vi "TSLIN_LIN_Schedule_add.vi"(8 "错误输入":errorcluster, 10 "LIN Scheduling Table Array":T1[](array[typedef]) {"LIN_Transmit"."FDatas"."value 7" format="%.0x"; "LIN_Transmit"."FDatas"."value 6" format="%.0x"; "LIN_Transmit"."FDatas"."value 5" format="%.0x"; "LIN_Transmit"."FDatas"."value 4" format="%.0x"; "LIN_Transmit"."FDatas"."value 3" format="%.0x"; "LIN_Transmit"."FDatas"."value 2" format="%.0x"; "LIN_Transmit"."FDatas"."value 1" format="%.0x"; "LIN_Transmit"."FDatas"."value0" format="%.0x"; "LIN_Transmit"."Channel" items=["CHN1", "CHN2", "CHN3", "CHN4", "CHN5", "CHN6", "CHN7", "CHN8", "CHN9", "CHN10", "CHN11", "CHN12", "CHN13", "CHN14", "CHN15", "CHN16", "CHN17", "CHN18", "CHN19", "CHN20", "CHN21", "CHN22", "CHN23", "CHN24", "CHN25", "CHN26", "CHN27", "CHN28", "CHN29", "CHN30", "CHN31", "CHN32"]; "LIN_Transmit"."ID" format="%.0x"; "LIN_Transmit"."DLC" format="%.0x"; "LIN_Transmit"."Set_node_funtiontype" items=["MasterNode", "SlaveNode", "MonitorNote"]}, 11 "路径输入":path) -> (0 "错误输出":errorcluster, 1 "Channel array":i32[](array[numeric]), 2 "Successful?":bool, 3 "路径输出":path)   [LabVIEW 2014]
uses:
  Typedef/TSLIN_Transmit.ctl
  Typedef/TSLIN_LIN Schedule_Table.ctl
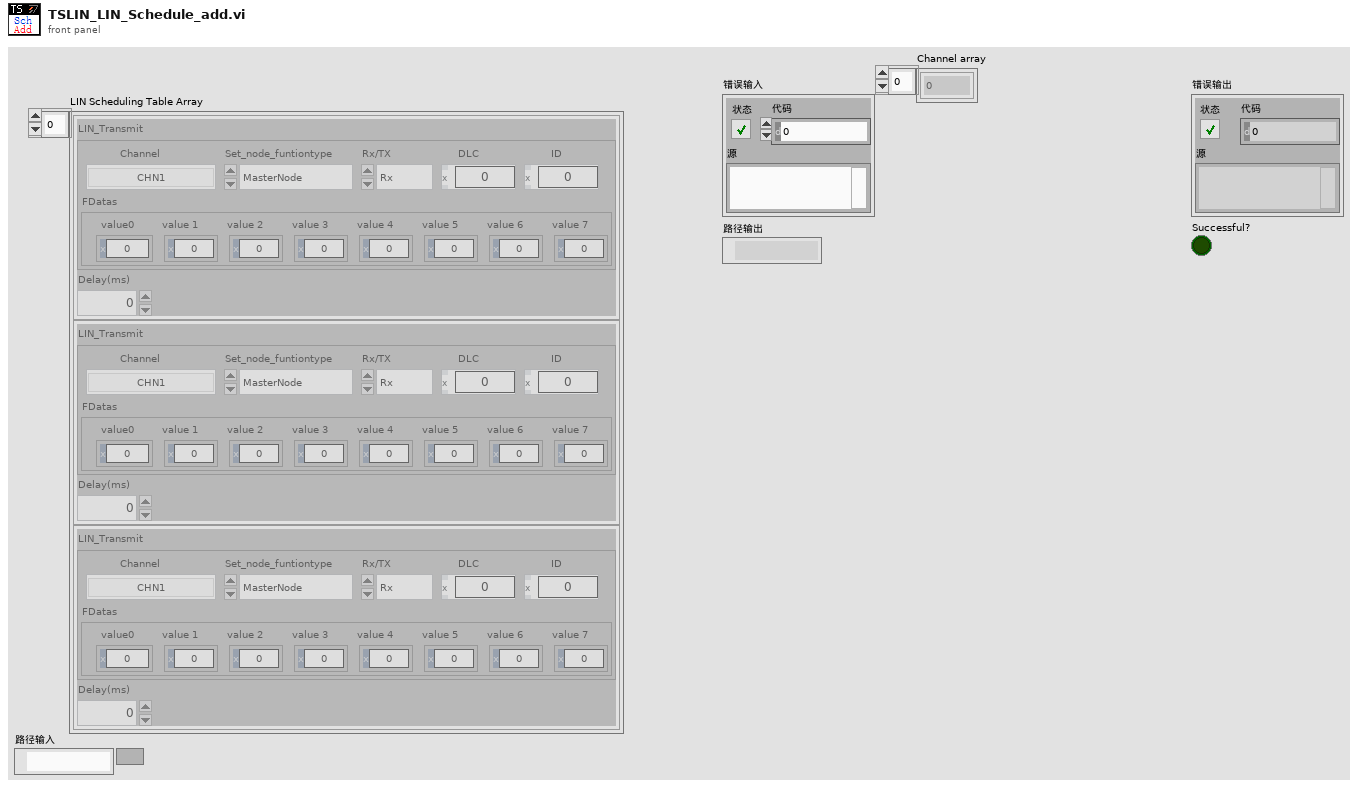
[diagram p1: front panel]
types:
  T1 = typedef "TSLIN_LIN Schedule_Table.ctl" = cluster{"LIN_Transmit":T2, "Delay(ms)":i32}
  T2 = typedef "TSLIN_Transmit.ctl" = cluster{"Channel":i32, "Rx/TX":enum16{"Rx", "Tx"}, "Set_node_funtiontype":i32, "DLC":u32, "ID":u32, "FDatas":cluster{"value0":u8, "value 1":u8, "value 2":u8, "value 3":u8, "value 4":u8, "value 5":u8, "value 6":u8, "value 7":u8}}
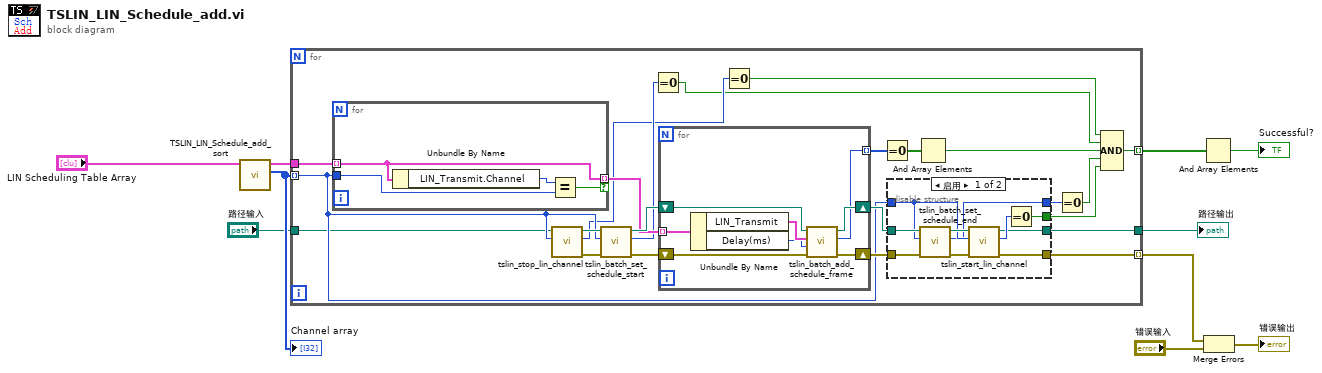
[diagram p0: block diagram]
diagram:
  n1 = call "TSLIN_LIN_Schedule_add_sort.vi"("LIN Scheduling Table Array"="LIN Scheduling Table Array") -> ("CH_array"=w8:i32[], "LIN Scheduling Table Array out"=w9:T1[])  [unwired: 9 in]
  "Channel array" <- w8
  n2 = for {
    tunnel: w9 -> [w33]
    tunnel: w8 -> [w26] mode=indexing
    tunnel: "路径输入" -> [w25]
    tunnel: [w23] -> w6 mode=indexing
    tunnel: [w12] -> w3 mode=indexing
    tunnel: [w11] -> w1
    n3 = for {
      tunnel: w33 -> [w55] mode=indexing
      tunnel: w26 -> [w56]
      tunnel: [w55] -> w24 mode=indexing if=w54
      n4 = Unbundle By Name(w55) -> ("LIN_Transmit.Channel"=w57:i32)
      n5 = Equal?(x=w57, y=w56) -> (x = y?=w54:bool)
    }
    n6 = call "tslin_stop_lin_channel.vi"("ALdxChn"=w26, "路径输入"=w25) -> ("错误输出"=w32:errorcluster, "return"=w18:i32, "路径输出"=w29:path)  [unwired: 7 in]
    n7 = call "tslin_batch_set_schedule_start.vi"("错误输入（无错误）"=w32, "AIdxChn"=w26, "路径输入"=w29) -> ("错误输出"=w31:errorcluster, "return"=w22:i32, "路径输出"=w28:path)  [unwired: 6 in]
    n8 = Equal To 0?(x=w22) -> (x = 0?=w16:bool)
    n9 = for {
      shift-right: [w52] -> w30
      shift-left: w31 -> [w53]
      shift-right: [w50] -> w27
      shift-left: w28 -> [w51]
      tunnel: w24 -> [w49] mode=indexing
      tunnel: [w46] -> w20 mode=indexing
      n10 = Unbundle By Name(w49) -> ("LIN_Transmit"=w48:T2, "Delay(ms)"=w47:i32)
      n11 = call "tslin_batch_add_schedule_frame.vi"("错误输入（无错误）"=w53, "ADelayMS"=w47, "LIN_Transmit"=w48, "路径输入"=w51) -> ("错误输出"=w52:errorcluster, "return"=w46:i32, "路径输出"=w50:path)  [unwired: 5 in]
    }
    n12 = Equal To 0?(x=w18) -> (x = 0?=w17:bool)
    n13 = Equal To 0?(x=w20) -> (x = 0?=w19:bool[])
    n14 = disable-structure shown="启用" {
      disable-tunnel: w30 -> [w42 w45]
      disable-tunnel: w27 -> [w41 w44]
      disable-tunnel: w26 -> [w39 _]
      disable-tunnel: [w38 w45] -> w23
      disable-tunnel: [w37 _] -> w21
      disable-tunnel: [w35 _] -> w13
      disable-tunnel: [w34 w44] -> w11
      frame Enabled {
        n15 = call "tslin_batch_set_schedule_end.vi"("错误输入（无错误）"=w42, "AIdxChn"=w39, "路径输入"=w41) -> ("错误输出"=w43:errorcluster, "return"=w37:i32, "路径输出"=w40:path)  [unwired: 6 in]
        n16 = call "tslin_start_lin_channel.vi"("错误输入（无错误）"=w43, "ALdxChn"=w39, "路径输入"=w40) -> ("错误输出"=w38:errorcluster, "return"=w36:i32, "路径输出"=w34:path)  [unwired: 6 in]
        n17 = Equal To 0?(x=w36) -> (x = 0?=w35:bool)
      }
      frame Disabled {
      }
    }
    n18 = And Array Elements(Boolean array=w19) -> (logical AND=w15:bool)
    n19 = Equal To 0?(x=w21) -> (x = 0?=w14:bool)
    n20 = Compound Arithmetic op=AND(w17, w16, w15, w14, w13) -> (w12:bool)
  }
  "路径输出" <- w1
  n21 = And Array Elements(Boolean array=w3) -> (logical AND=→"Successful?":bool)
  n22 = Merge Errors(w6, "错误输入") -> (→"错误输出":errorcluster)
